vi "Run_VI_Named_specific.vi"(8 "Run VI Named String":string, 10 "Earlier Filenames":path[](array[path]), 11 "Multi Run Row":T1 {"Carrier_2 Q (l/min)" format="%#.2f"; "Row Duration (mins)" format="%#.1f"; "Row No" min=0; "Trace Gas Concentration (%)" min=0.0 format="%#_4f"; "Carrier_1 Q (l/min)" format="%#.2f"; "Tunnel Speed" format="%#.2f"; "Start X" format="%#.2f"; "Start Y" format="%#.2f"; "Start Z" format="%#.2f"; "End X" format="%#.2f"; "End Y" format="%#.2f"; "End Z" format="%#.2f"; "Averaging time (min)" min=0.0 format="%#.2f"}) -> (0 "Scalable Time (Sec)":dbl format="%.2f", 1 "Fixed Time (Sec)":dbl format="%.2f", 2 "Channel Names":string[](array[string]), 3 "Checks":string[](array[string]), 4 "Error String":string, 5 "Check Meas Setup?":bool, 6 "Check for start NaNs?":bool)   [LabVIEW 2015]
uses:
  Gen Trav/Traverse_cluster.ctl
  Gen Trav/Spacing.ctl
  Controls/Multi_run_mode.ctl
  Globals/Preference_global.vi
panel:
  # "X           Y            Z"
  # "Start"
  # "End"
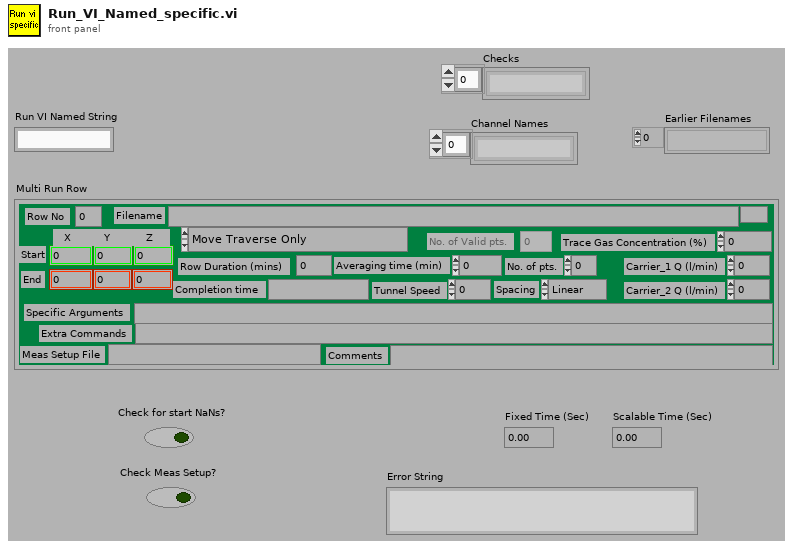
[diagram p1: front panel]
types:
  T1 = typedef "Traverse_cluster.ctl" = cluster{"Start X":sgl, "Start Y":sgl, "Start Z":sgl, "End X":sgl, "End Y":sgl, "End Z":sgl, "No. of pts.":i32, "Spacing":T2, "Filename":path, "Tunnel Speed":dbl, "Averaging time (min)":dbl, "Extra Commands":string, "Carrier_1 Q (l/min)":dbl, "Carrier_2 Q (l/min)":dbl, "Trace Gas Concentration (%)":dbl, "Specific Arguments":string, "Comments":string, "Row No":i32, "Row Type Selector":T3, "Completion time":string, "Row Duration (mins)":dbl, "No. of Valid pts.":i32, "Meas Setup File":string}
  T2 = typedef "Spacing.ctl" = enum16{"Linear", "Log", "Gauss", "Specified", "N/A"}
  T3 = typedef "Multi_run_mode.ctl" = enum16{"Move Traverse Only", "Set Tunnel Speed Only", "Set Source Only", "Set Measurement Conditions", "Single Measurement", "Vertical Profile", "Lateral Profile", "Longitudinal Profile", "Explore Volume", "Multi-Axis Profile", "Auto Calibrate", "Meas Fast FID Bkgnd", "Check Beam Power", "Scanning Valve Measurement", "Run VI Named:", "Set ADAM Ch", "Wait (minutes)", "Send Message", "Synchronize With:", "Fall Back to this Row", "Turn Off Row Repeating", "Blank Row", "Traverse 3D Volume"}
  T4 = typedef "Beam_Type.ctl" = u16
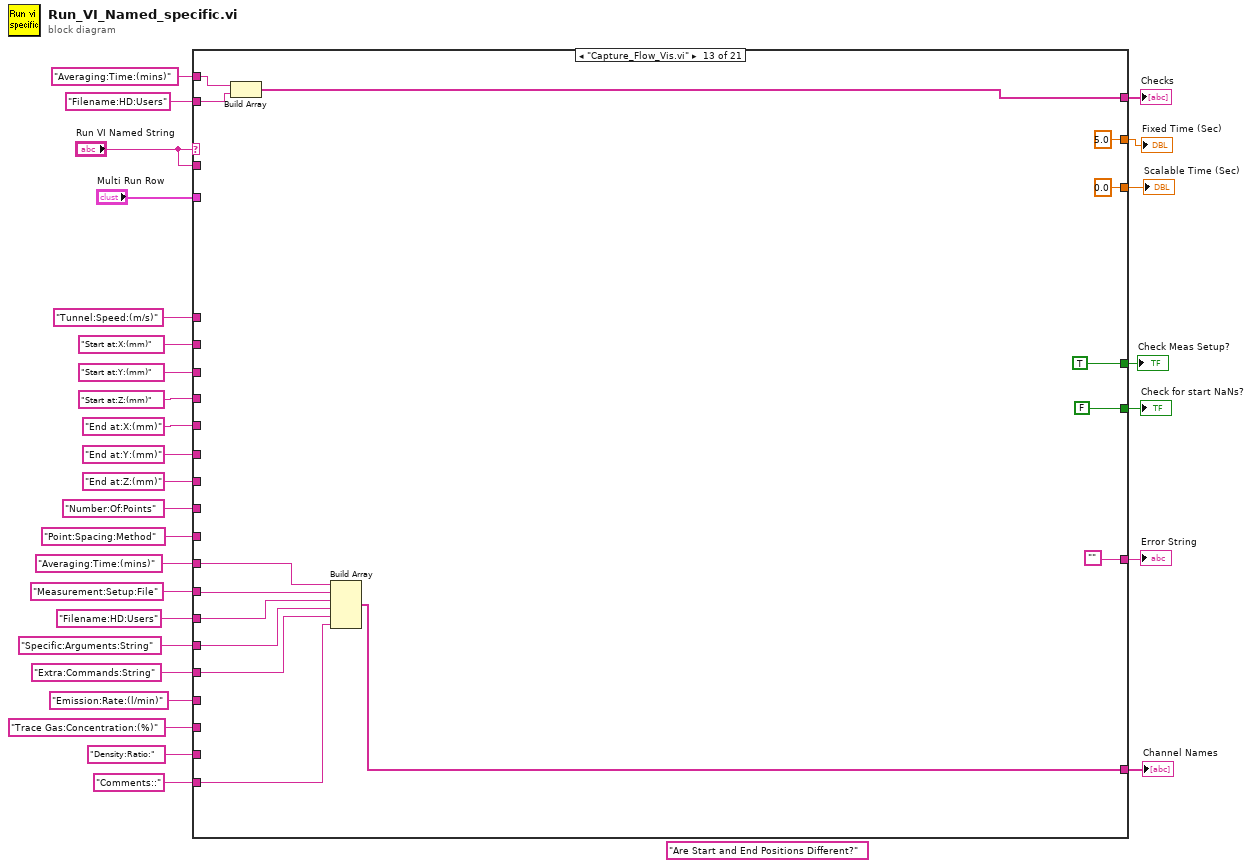
[diagram p0: block diagram]
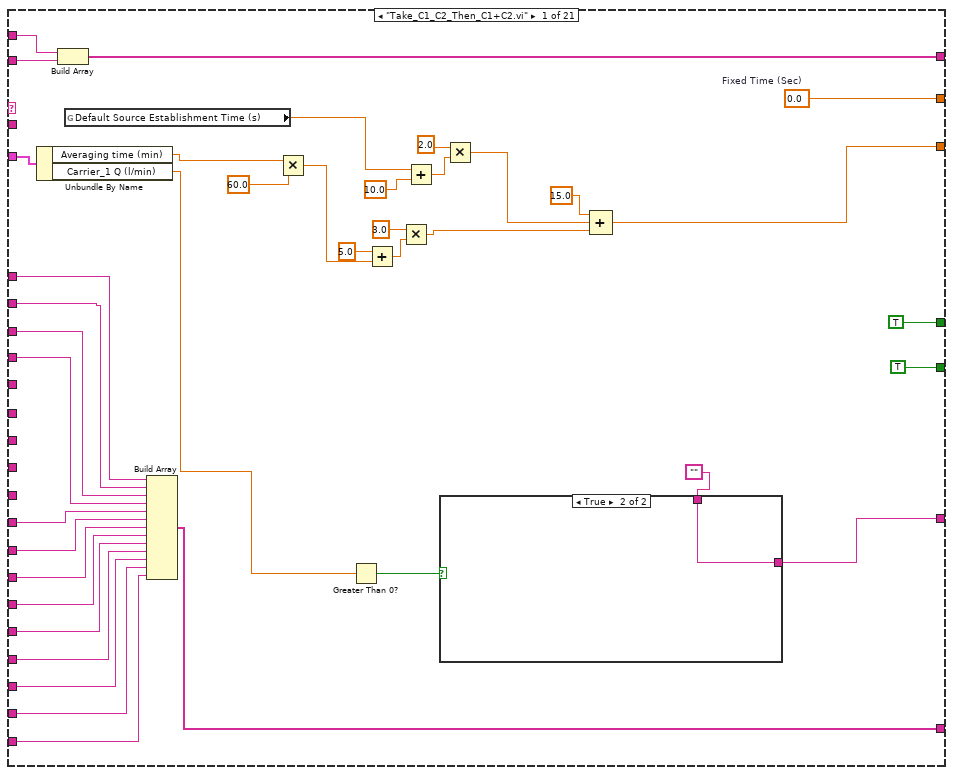
[diagram p2: hidden frame]
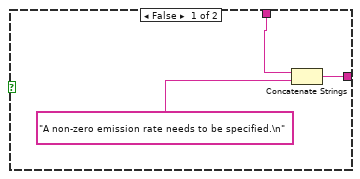
[diagram p3: hidden frame]
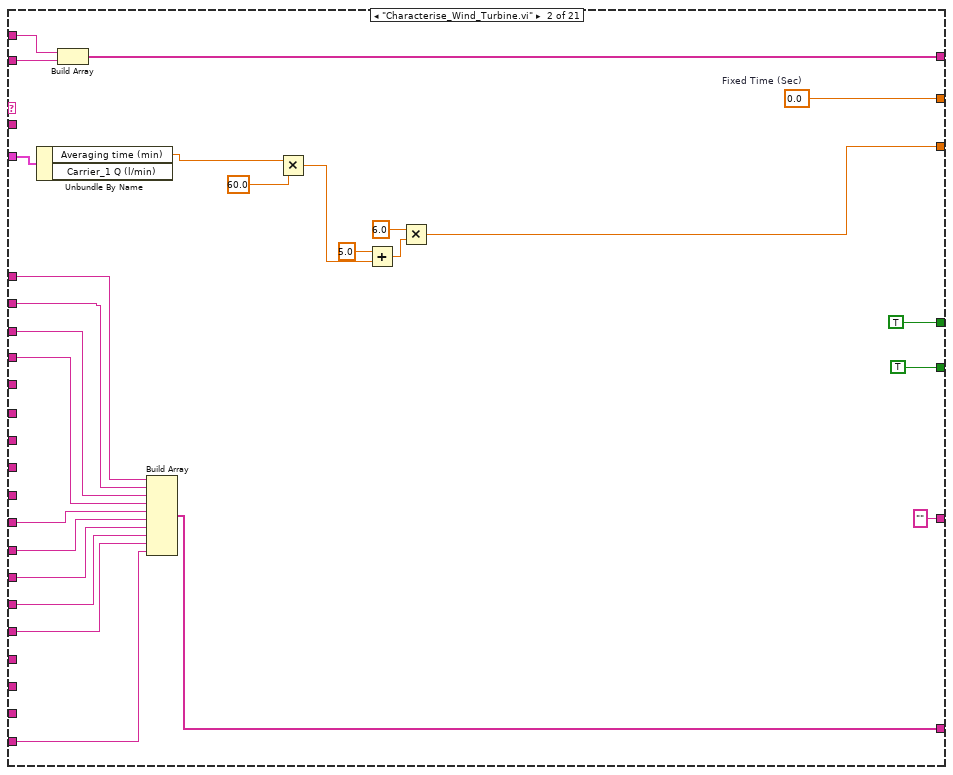
[diagram p4: hidden frame]
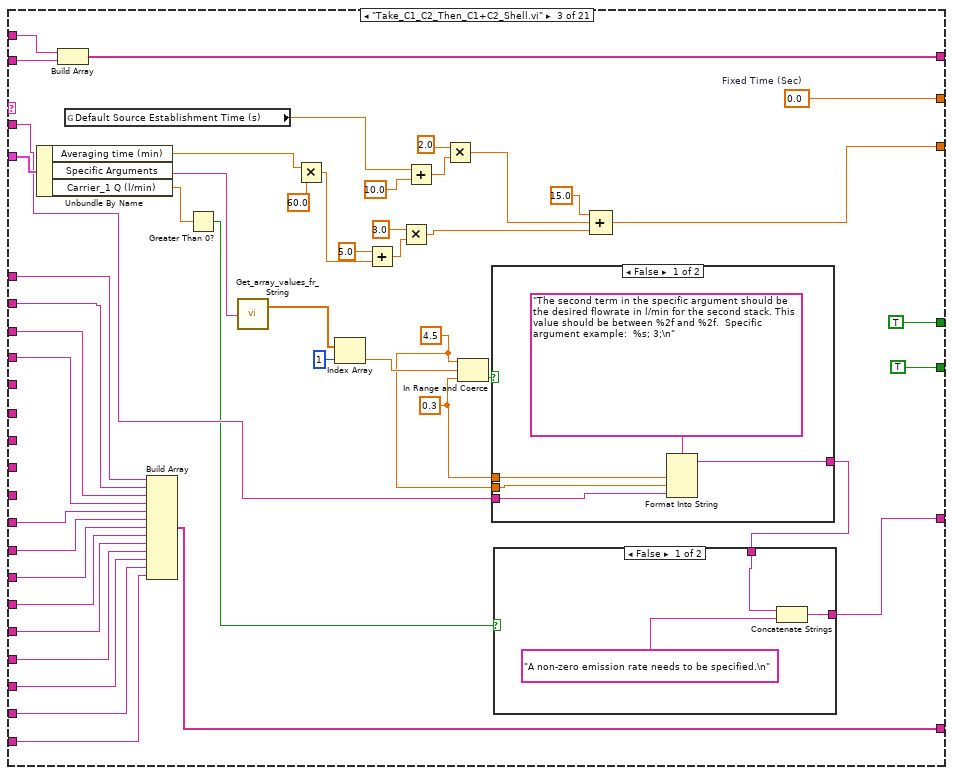
[diagram p5: hidden frame]
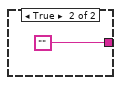
[diagram p7: hidden frame]
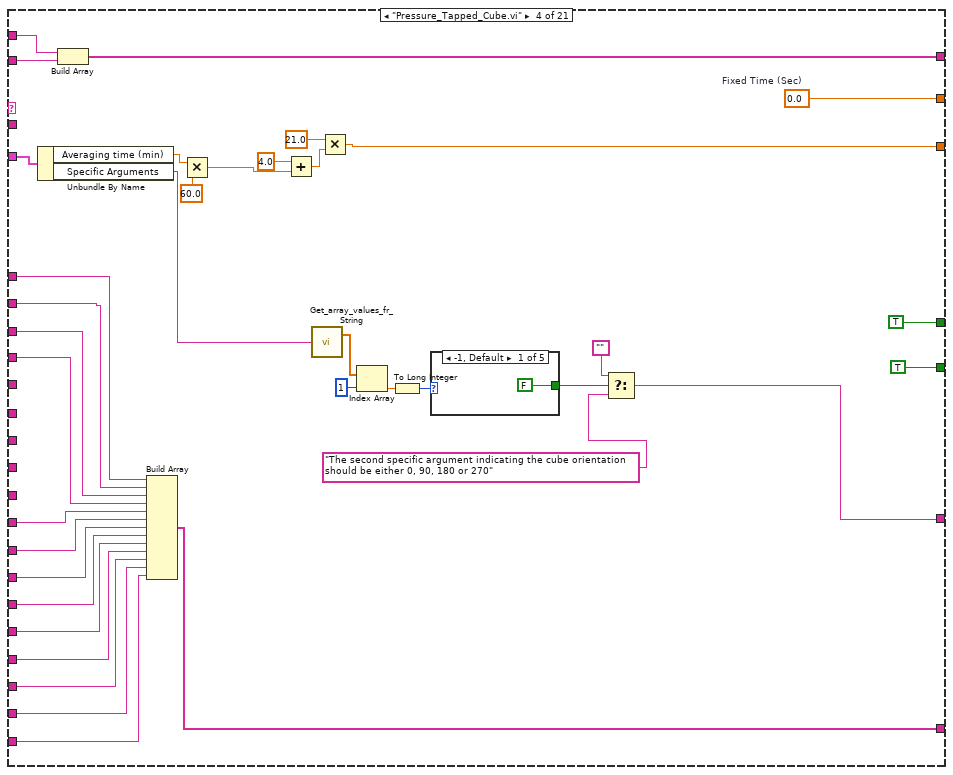
[diagram p8: hidden frame]
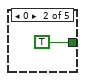
[diagram p9: hidden frame]
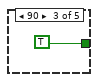
[diagram p10: hidden frame]
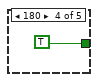
[diagram p11: hidden frame]
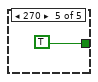
[diagram p12: hidden frame]
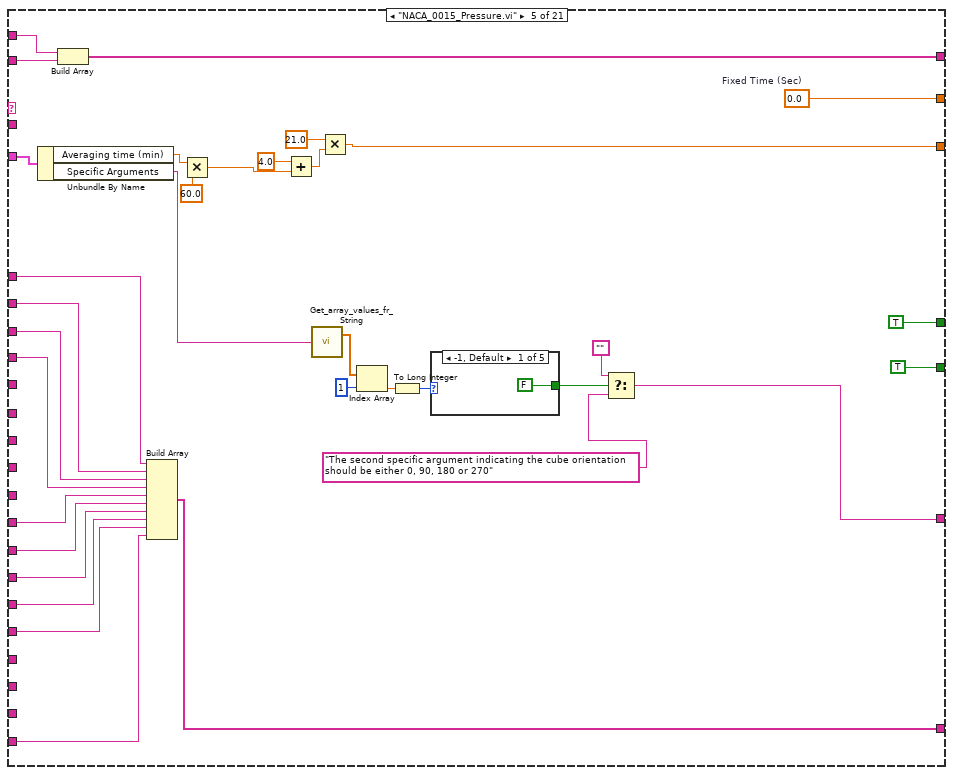
[diagram p13: hidden frame]
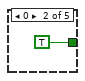
[diagram p14: hidden frame]
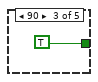
[diagram p15: hidden frame]
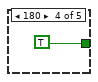
[diagram p16: hidden frame]
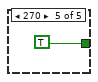
[diagram p17: hidden frame]
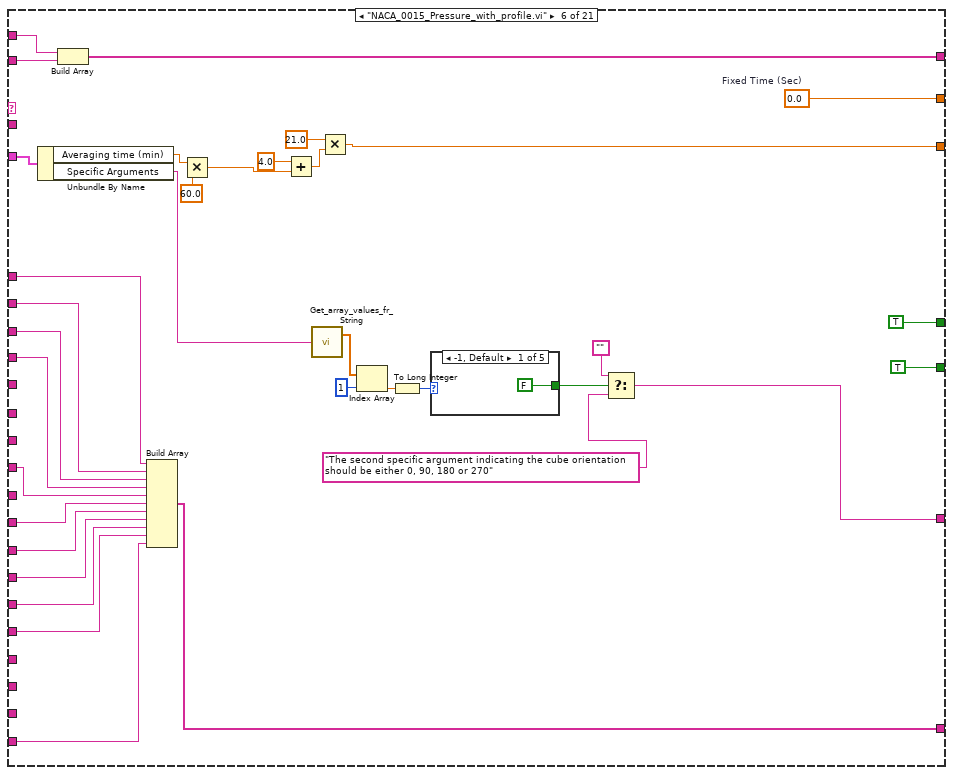
[diagram p18: hidden frame]
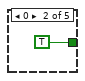
[diagram p19: hidden frame]
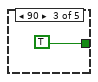
[diagram p20: hidden frame]
diagram:
  (unwired) "Are Start and End Positions Different?" ("Label for value")
  n1 = case shown="\"Capture_Flow_Vis.vi\"" "Run VI Named String" {
    tunnel: "Multi Run Row" -> [w68 w98 w145 w192 w231 w271 w314 w321 _ w376 _ _ _ _ w456 w480 _ _ w527 w556 w582]
    tunnel: [w67 w97 w144 w191 w230 w270 w313 w355 w371 w386 0.0 ("Fixed Time (Sec)") 5.0 ("Fixed Time (Sec)") 5.0 ("Fixed Time (Sec)") 5.0 ("Fixed Time (Sec)") 5.0 ("Fixed Time (Sec)") 5.0 ("Fixed Time (Sec)") 40.0 ("Fixed Time (Sec)") 40.0 ("Fixed Time (Sec)") w521 w548 w581] -> w28
    tunnel: [w53 w74 w130 w165 w210 w250 w295 w319 60.0 ("value") 0.0 ("value") 6.0 ("value") 0.0 ("value") 0.0 ("value") 0.0 ("value") 0.0 ("value") 0.0 ("value") 0.0 ("value") 0.0 ("value") w522 w555 40.0 ("value")] -> w27
    tunnel: "Averaging:Time:(mins)" ("Label for value") -> [w52 w90 w129 w188 w227 w267 w310 w353 w370 _ _ _ w428 _ _ _ _ _ _ _ _]
    tunnel: "Filename:HD:Users" ("Label for value") -> [w51 w89 w128 w187 w226 w266 w309 w352 w369 _ _ _ w426 _ _ _ _ _ _ _ _]
    tunnel: [TRUE TRUE TRUE TRUE TRUE TRUE FALSE TRUE TRUE FALSE FALSE FALSE FALSE FALSE FALSE FALSE FALSE FALSE FALSE FALSE TRUE] -> w24
    tunnel: [TRUE TRUE TRUE TRUE TRUE TRUE TRUE TRUE TRUE FALSE FALSE FALSE TRUE FALSE FALSE FALSE FALSE FALSE FALSE TRUE FALSE] -> w23
    tunnel: [w48 w86 w125 w184 w223 w263 w306 w349 w366 string[] [] string[] [] string[] [] w427 string[] [] string[] [] string[] [] string[] [] string[] [] string[] [] string[] [] string[] []] -> w22
    tunnel: "Tunnel:Speed:(m/s)" ("Label for value") -> [w47 w85 w124 w183 w200 w240 _ w348 _ w377 w400 _ _ _ _ _ _ _ _ w535 _]
    tunnel: "Start at:X:(mm)" ("Label for value") -> [w46 w84 w123 w182 w199 w239 _ w347 w365 _ w409 _ _ _ _ w478 w497 w505 _ _ w578]
    tunnel: "Start at:Y:(mm)" ("Label for value") -> [w45 w83 w122 w181 w198 w238 _ w346 w364 _ w408 _ _ _ _ w477 _ w508 _ _ w577]
    tunnel: "Start at:Z:(mm)" ("Label for value") -> [w44 w82 w121 w180 w222 w262 _ w345 w363 _ w407 _ _ _ _ w476 _ _ _ _ w576]
    tunnel: "Averaging:Time:(mins)" ("Label for value") -> [w43 w81 w120 w179 w221 w261 w291 w344 _ _ w399 _ w430 _ _ _ _ _ _ w544 _]
    tunnel: "Measurement:Setup:File" ("Label for value") -> [w42 w80 w119 w178 w220 w260 w305 w343 w362 _ w395 _ w431 _ _ _ w493 w509 _ w545 _]
    tunnel: "Filename:HD:Users" ("Label for value") -> [w41 w79 w118 w177 w219 w259 w304 w342 _ _ w401 _ w429 _ w457 w474 _ _ _ w546 _]
    tunnel: "Specific:Arguments:String" ("Label for value") -> [w40 w78 w117 w176 w218 w258 w303 w341 w361 w383 w394 w423 w438 w448 w464 w475 w494 w510 w532 w547 w564]
    tunnel: "Extra:Commands:String" ("Label for value") -> [w39 w77 w116 w175 w217 w257 w302 w340 w360 w382 w393 w422 w437 w447 w463 w488 w495 w511 w531 w560 w563]
    tunnel: "Emission:Rate:(l/min)" ("Label for value") -> [w38 _ w115 w174 _ _ _ w339 _ _ w398 _ _ _ _ _ _ _ _ _ _]
    tunnel: "Trace Gas:Concentration:(%)" ("Label for value") -> [w37 _ w114 w173 _ _ _ w338 _ _ w397 _ _ _ _ _ _ _ _ _ _]
    tunnel: "Density:Ratio:" ("Label for value") -> [w36 _ w113 w172 _ _ _ w337 _ _ w396 _ _ _ _ _ _ _ _ _ _]
    tunnel: "Comments::" ("Label for value") -> [w35 w76 w112 w171 w216 w256 w301 w336 w359 w381 w392 w421 w436 w446 w462 w487 w496 w512 w530 w559 w572]
    tunnel: [w34 w75 w111 w170 w215 w255 w300 w335 w358 w380 w391 w420 w435 w445 w461 w486 w502 w517 w529 w558 w575] -> w8
    tunnel: [w32 "" ("Error Comments") w99 w156 w201 w241 w293 w318 "" w372 "" "" "" "" w452 "" "" "" w520 w550 w566] -> w7
    tunnel: "End at:X:(mm)" ("Label for value") -> [_ _ _ _ _ _ _ w317 _ _ w406 _ _ _ _ _ _ w507 _ _ w573]
    tunnel: "End at:Y:(mm)" ("Label for value") -> [_ _ _ _ _ _ _ w316 _ _ w405 _ _ _ _ _ _ w506 _ _ _]
    tunnel: "End at:Z:(mm)" ("Label for value") -> [_ _ _ _ _ _ _ w315 _ _ w404 _ _ _ _ _ _ _ _ _ _]
    tunnel: "Run VI Named String" -> [_ _ w105 _ _ _ _ _ _ _ _ _ _ _ _ _ _ _ _ _ _]
    tunnel: "Number:Of:Points" ("Label for value") -> [_ _ _ _ _ w237 w292 _ _ _ w403 _ _ _ _ _ _ _ _ _ _]
    tunnel: "Point:Spacing:Method" ("Label for value") -> [_ _ _ _ _ _ w290 _ _ _ w402 _ _ _ _ _ _ _ _ _ _]
    frame "Take_C1_C2_Then_C1+C2.vi" {
      w67 = 0.0  # Fixed Time (Sec)
      n2 = Unbundle By Name(w68) -> ("Averaging time (min)"=w56:dbl, "Carrier_1 Q (l/min)"=w31:dbl)
      n3 = Build Array(w52, w51) -> (w48:string[])
      n4 = global read "Preference_global.vi" "Default Source Establishment Time (s)"() -> (w57:dbl)
      n5 = Build Array(w47, w46, w45, w44, w43, w42, w41, w40, w39, w38, w37, w36, w35) -> (w34:string[])
      n6 = Multiply(x=w56, y=60.0) -> (x*y=w54:dbl)
      n7 = Greater Than 0?(x=w31) -> (x > 0?=w30:bool)
      n8 = Add(x=5.0, y=w54) -> (x+y=w60:dbl)
      n9 = Multiply(x=3.0, y=w60) -> (x*y=w64:dbl)
      n10 = Add(x=w57, y=10.0) -> (x+y=w62:dbl)
      n11 = case shown="True" w30 {
        tunnel: "" -> [w70 w72]
        tunnel: [w69 w72] -> w32
        frame False {
          n12 = Concatenate Strings(w70, "A non-zero emission rate needs to be specified.\n") -> (w69:string)
        }
        frame True {
        }
      }
      n13 = Multiply(x=2.0, y=w62) -> (x*y=w65:dbl)
      n14 = Compound Arithmetic op=ADD(15.0 ("value"), w65, w64) -> (w53:dbl)
    }
    frame "Characterise_Wind_Turbine.vi" {
      w97 = 0.0  # Fixed Time (Sec)
      n15 = Unbundle By Name(w98) -> ("Averaging time (min)"=w93:dbl)  [unwired: 1 out]
      n16 = Build Array(w90, w89) -> (w86:string[])
      n17 = Build Array(w85, w84, w83, w82, w81, w80, w79, w78, w77, w76) -> (w75:string[])
      n18 = Multiply(x=w93, y=60.0) -> (x*y=w91:dbl)
      n19 = Add(x=5.0, y=w91) -> (x+y=w96:dbl)
      n20 = Multiply(x=6.0, y=w96) -> (x*y=w74:dbl)
    }
    frame "Take_C1_C2_Then_C1+C2_Shell.vi" {
      w103 = 4.5 ("upper limit")
      w104 = 0.3 ("lower limit")
      w144 = 0.0  # Fixed Time (Sec)
      n21 = Unbundle By Name(w145) -> ("Averaging time (min)"=w133:dbl, "Specific Arguments"=w108:string, "Carrier_1 Q (l/min)"=w102:dbl)
      n22 = Build Array(w129, w128) -> (w125:string[])
      n23 = global read "Preference_global.vi" "Default Source Establishment Time (s)"() -> (w134:dbl)
      n24 = Build Array(w124, w123, w122, w121, w120, w119, w118, w117, w116, w115, w114, w113, w112) -> (w111:string[])
      n25 = Greater Than 0?(x=w102) -> (x > 0?=w101:bool)
      n26 = call "Get_array_values_fr_String.vi"("String Value"=w108) -> ("Numeric Array"=w110:dbl[])  [unwired: 1 out]
      n27 = Multiply(x=w133, y=60.0) -> (x*y=w131:dbl)
      n28 = Index Array(array=w110, index=1) -> (element=w107:dbl)
      n29 = Add(x=5.0, y=w131) -> (x+y=w137:dbl)
      n30 = Multiply(x=3.0, y=w137) -> (x*y=w141:dbl)
      n31 = Add(x=w134, y=10.0) -> (x+y=w139:dbl)
      n32 = Multiply(x=2.0, y=w139) -> (x*y=w142:dbl)
      n33 = In Range and Coerce(upper limit=w103, x=w107, lower limit=w104) -> (In Range?=w106:bool)  [unwired: 1 out]
      n34 = case shown="False" w106 {
        tunnel: [w150 ""] -> w100
        tunnel: w105 -> [w154 _]
        tunnel: w104 -> [w153 _]
        tunnel: w103 -> [w152 _]
        frame False {
          n35 = Format Into String(format string="The second term in the specific argument should be the desired flowrate in l/min for the second stack. This value should be between %2f and %2f.  Specific argument example:  %s; 3;\n", w153, w152, w154) -> (resulting string=w150:string)  [unwired: 2 in, 1 out]
        }
        frame True {
        }
      }
      n36 = case shown="False" w101 {
        tunnel: w100 -> [w147 w149]
        tunnel: [w146 w149] -> w99
        frame False {
          n37 = Concatenate Strings(w147, "A non-zero emission rate needs to be specified.\n") -> (w146:string)
        }
        frame True {
        }
      }
      n38 = Compound Arithmetic op=ADD(15.0 ("value"), w142, w141) -> (w130:dbl)
    }
    frame "Pressure_Tapped_Cube.vi" {
      w191 = 0.0  # Fixed Time (Sec)
      n39 = Unbundle By Name(w192) -> ("Averaging time (min)"=w190:dbl, "Specific Arguments"=w157:string)
      n40 = Build Array(w188, w187) -> (w184:string[])
      n41 = Build Array(w183, w182, w181, w180, w179, w178, w177, w176, w175, w174, w173, w172, w171) -> (w170:string[])
      n42 = Multiply(x=w190, y=60.0) -> (x*y=w166:dbl)
      n43 = Add(x=4.0, y=w166) -> (x+y=w169:dbl)
      n44 = call "Get_array_values_fr_String.vi"("String Value"=w157) -> ("Numeric Array"=w159:dbl[])  [unwired: 1 out]
      n45 = Multiply(x=21.0, y=w169) -> (x*y=w165:dbl)
      n46 = Index Array(array=w159, index=1) -> (element=w160:dbl)
      n47 = To Long Integer(number=w160) -> (32bit integer=w161:i32)
      n48 = case shown="-1, Default" w161 {
        tunnel: [FALSE TRUE TRUE TRUE TRUE] -> w164
        frame -1, Default {
        }
        frame 0 {
        }
        frame 90 {
        }
        frame 180 {
        }
        frame 270 {
        }
      }
      n49 = Select(t="", s=w164, f="The second specific argument indicating the cube orientation should be either 0, 90, 180 or 270") -> (s? t:f=w156:string)
    }
    frame "NACA_0015_Pressure.vi" {
      w230 = 0.0  # Fixed Time (Sec)
      n50 = Unbundle By Name(w231) -> ("Averaging time (min)"=w229:dbl, "Specific Arguments"=w202:string)
      n51 = Build Array(w227, w226) -> (w223:string[])
      n52 = Build Array(w200, w199, w198, w222, w221, w220, w219, w218, w217, w216) -> (w215:string[])
      n53 = Multiply(x=w229, y=60.0) -> (x*y=w211:dbl)
      n54 = Add(x=4.0, y=w211) -> (x+y=w214:dbl)
      n55 = call "Get_array_values_fr_String.vi"("String Value"=w202) -> ("Numeric Array"=w204:dbl[])  [unwired: 1 out]
      n56 = Multiply(x=21.0, y=w214) -> (x*y=w210:dbl)
      n57 = Index Array(array=w204, index=1) -> (element=w205:dbl)
      n58 = To Long Integer(number=w205) -> (32bit integer=w206:i32)
      n59 = case shown="-1, Default" w206 {
        tunnel: [FALSE TRUE TRUE TRUE TRUE] -> w209
        frame -1, Default {
        }
        frame 0 {
        }
        frame 90 {
        }
        frame 180 {
        }
        frame 270 {
        }
      }
      n60 = Select(t="", s=w209, f="The second specific argument indicating the cube orientation should be either 0, 90, 180 or 270") -> (s? t:f=w201:string)
    }
    frame "NACA_0015_Pressure_with_profile.vi" {
      w270 = 0.0  # Fixed Time (Sec)
      n61 = Unbundle By Name(w271) -> ("Averaging time (min)"=w269:dbl, "Specific Arguments"=w242:string)
      n62 = Build Array(w267, w266) -> (w263:string[])
      n63 = Build Array(w240, w239, w238, w262, w237, w261, w260, w259, w258, w257, w256) -> (w255:string[])
      n64 = Multiply(x=w269, y=60.0) -> (x*y=w251:dbl)
      n65 = Add(x=4.0, y=w251) -> (x+y=w254:dbl)
      n66 = call "Get_array_values_fr_String.vi"("String Value"=w242) -> ("Numeric Array"=w244:dbl[])  [unwired: 1 out]
      n67 = Multiply(x=21.0, y=w254) -> (x*y=w250:dbl)
      n68 = Index Array(array=w244, index=1) -> (element=w245:dbl)
      n69 = To Long Integer(number=w245) -> (32bit integer=w246:i32)
      n70 = case shown="-1, Default" w246 {
        tunnel: [FALSE TRUE TRUE TRUE TRUE] -> w249
        frame -1, Default {
        }
        frame 0 {
        }
        frame 90 {
        }
        frame 180 {
        }
        frame 270 {
        }
      }
      n71 = Select(t="", s=w249, f="The second specific argument indicating the cube orientation should be either 0, 90, 180 or 270") -> (s? t:f=w241:string)
    }
    frame "Measure_Synthetic_Jet.vi" {
      w313 = 0.0  # Fixed Time (Sec)
      n72 = Unbundle By Name(w314) -> ("Averaging time (min)"=w312:dbl, "Specific Arguments"=w294:string)
      n73 = Build Array(w310, w309) -> (w306:string[])
      n74 = Build Array(w292, w290, w291, w305, w304, w303, w302, w301) -> (w300:string[])
      n75 = Multiply(x=w312, y=60.0) -> (x*y=w296:dbl)
      n76 = Add(x=4.0, y=w296) -> (x+y=w299:dbl)
      n77 = call "Get_array_values_fr_String.vi"("String Value"=w294) -> ("String array"=w289:string[])  [unwired: 1 out]
      n78 = Multiply(x=21.0, y=w299) -> (x*y=w295:dbl)
      n79 = Index Array(array=w289, index #1=1 ("index")) -> (element #1=w284:string, element #2=w282:string, element #3=w281:string, element #4=w278:string)  [unwired: 3 in]
      n80 = Empty String/Path?(string/path=w278) -> (empty?=w277:bool)
      n81 = Empty String/Path?(string/path=w282) -> (empty?=w279:bool)
      n82 = Empty String/Path?(string/path=w284) -> (empty?=w283:bool)
      n83 = Empty String/Path?(string/path=w281) -> (empty?=w280:bool)
      n84 = Compound Arithmetic op=OR(w283, w279, w280, w277) -> (w287:bool)
      n85 = Select(t="The second, third and fourth specific argument indicate the min frequency, max frequency, the number of bins to use in the phase average and the target amplitude.  Set the target optimisation target value to -1 if you do not want any optimisation. Example: Measure_Synthetic_Jet.vi; 100; 1000; 50; 0.02", s=w287, f="") -> (s? t:f=w293:string)
    }
    frame "Take_Data_on_the_Move.vi" {
      w355 = 0.0  # Fixed Time (Sec)
      n86 = Build Array(w353, w352) -> (w349:string[])
      n87 = Build Array(w348, w347, w346, w345, w317, w316, w315, w344, w343, w342, w341, w340, w339, w338, w337, w336) -> (w335:string[])
      n88 = Unbundle By Name(w321) -> ("Averaging time (min)"=w320:dbl, "Start X"=w322:sgl, "Start Y"=w323:sgl, "Start Z"=w324:sgl, "End X"=w325:sgl, "End Y"=w326:sgl, "End Z"=w327:sgl)
      n89 = Build Array(w322, w323, w324) -> (w329:sgl[])
      n90 = Build Array(w325, w326, w327) -> (w328:sgl[])
      n91 = Multiply(x=w320, y=60.0) -> (x*y=w333:dbl)
      n92 = Not Equal?(x=w329, y=w328) -> (x != y?=w332:bool)
      n93 = Select(t="", s=w332, f="The Start and End positions must not be the same.\n" ("Format String")) -> (s? t:f=w318:string)
      n94 = Add(x=10.0, y=w333) -> (x+y=w319:dbl)
    }
    frame "Check_FID_Response.vi" {
      w371 = 0.0  # Fixed Time (Sec)
      n95 = Build Array(w370, w369) -> (w366:string[])
      n96 = Build Array(w365, w364, w363, w362, w361, w360, w359) -> (w358:string[])
    }
    frame "Return_EnFlo_Tunnel_to_Neutral.vi" {
      w373 = 0.4 ("y")
      w386 = 240.0  # Fixed Time (Sec)
      n97 = Unbundle By Name(w376) -> ("Tunnel Speed"=w375:dbl)
      n98 = Build Array(w377, w383, w382, w381) -> (w380:string[])
      n99 = Greater?(x=w375, y=w373) -> (0:w374:bool)
      n100 = case shown="True" w374 {
        tunnel: w373 -> [w389 _]
        tunnel: [w387 ""] -> w372
        frame False {
          n101 = Format Into String(format string="The Tunnel speed must be greater than %.1f", w389) -> (resulting string=w387:string)  [unwired: 2 in, 1 out]
        }
        frame True {
        }
      }
    }
    frame "No Match", Default {
      n102 = Build Array(w409, w408, w407, w406, w405, w404, w403, w402, w401, w400, w399, w393, w394, w398, w397, w396, w392, w395) -> (w391:string[])
    }
    frame "Set_Wind_Turbine_Speed.vi" {
      n103 = Build Array(w423, w422, w421) -> (w420:string[])
    }
    frame "Capture_Flow_Vis.vi" {
      n104 = Build Array(w428, w426) -> (w427:string[])
      n105 = Build Array(w430, w431, w429, w438, w437, w436) -> (w435:string[])
    }
    frame "Shut_down_EnFlo_Tunnel.vi" {
      n106 = Build Array(w448, w447, w446) -> (w445:string[])
    }
    frame "Update_Inlet_Temp_Profile.vi" {
      n107 = Unbundle By Name(w456) -> ("Filename"=w451:path)
      n108 = Build Array(w457, w464, w463, w462) -> (w461:string[])
      n109 = Search 1D Array(1D array="Earlier Filenames", element=w451) -> (index of element=w454:i32)  [unwired: 1 in]
      n110 = case shown="0, Default" w454 {
        tunnel: w451 -> [_ w473]
        tunnel: [TRUE ("exists?") w472] -> w453
        frame 0, Default {
        }
        frame -1 {
          n111 = call "Does_file_exist_(simple).vi"("Pathname"=w473) -> ("exists?"=w472:bool)
        }
      }
      n112 = case shown="False" w453 {
        tunnel: [w467 ""] -> w452
        tunnel: w451 -> [w469 _]
        frame False {
          n113 = Format Into String(format string="Cannot find Filename%s", w469) -> (resulting string=w467:string)  [unwired: 2 in, 1 out]
        }
        frame True {
        }
      }
    }
    frame "Datum_Image_Calibration.vi" {
      n114 = Unbundle By Name(w480) -> ("Filename"=w479:path)
      n115 = Build Array(w478, w477, w476, w474, w475, w488, w487) -> (w486:string[])
      n116 = call "Does_file_exist_(simple).vi"("Pathname"=w479) -> ("exists?"=w481:bool)
      n117 = case shown="False" w481 {
        tunnel: w479 -> [w492 _]
        frame False {
          n118 = Write to Text File(file (use dialog)=w492, text="Created so that multirun checker is happy that the file exists") -> ()  [unwired: 2 in, 3 out]
        }
        frame True {
        }
      }
    }
    frame "EnFlo_Turntable_Control.vi" {
      n119 = Build Array(w497, w493, w494, w495, w496) -> (w502:string[])
    }
    frame "Plot_Rectangle.vi" {
      n120 = Build Array(w505, w508, w507, w506, w509, w510, w511, w512) -> (w517:string[])
    }
    frame "Find_Beam_Max_Pos.vi" {
      w526 = 240.0  # Fixed Time (Sec)
      w522 = 0.0  # Scalable Time (Sec)
      n121 = Unbundle By Name(w527) -> ("Specific Arguments"=w523:string)
      n122 = Build Array(w532, w531, w530) -> (w529:string[])
      n123 = call "Get_Beam_names.vi"("String Value"=w523) -> ("Beam Array"=w524:T4[], "Error Comments"=w520:string)  [unwired: 1 out]
      n124 = Array Size(array=w524) -> (size(s)=w525:i32)
      n125 = Multiply(x=w526, y=w525) -> (x*y=w521:dbl)
    }
    frame "Find_Max_Value.vi" {
      w548 = 240.0  # Fixed Time (Sec)
      w555 = 0.0  # Scalable Time (Sec)
      n126 = Unbundle By Name(w556) -> ("Specific Arguments"=w553:string)
      n127 = Build Array(w535, w544, w545, w546, w547, w560, w559) -> (w558:string[])
      n128 = call "Get_array_values_fr_String.vi"("String Value"=w553) -> ("String array"=w554:string[])  [unwired: 1 out]
      n129 = Index Array(array=w554) -> (element #2=w552:string, element #3=w543:string, element #4=w537:string, element #5=w536:string)  [unwired: 5 in, 1 out]
      n130 = Empty String/Path?(string/path=w536) -> (empty?=w539:bool)
      n131 = Empty String/Path?(string/path=w552) -> (empty?=w542:bool)
      n132 = Empty String/Path?(string/path=w543) -> (empty?=w541:bool)
      n133 = Empty String/Path?(string/path=w537) -> (empty?=w538:bool)
      n134 = Compound Arithmetic op=OR(w542, w541, w538, w539) -> (w540:bool)
      n135 = Select(t="The second argument should be contain the fixed axis, followed by the search step in mm, the measurement channel to use for the survey and finally the data type you would like to measure, for example: Z Axis; 0.75; 2; uw/u'w'", s=w540, f="" ("Error Comments")) -> (s? t:f=w550:string)
    }
    frame "Move_Twin_Stacks.vi" {
      w581 = 0.0  # Fixed Time (Sec)
      n136 = Unbundle By Name(w582) -> ("End X"=w569:sgl)
      n137 = Build Array(w578, w577, w576, w573, w564, w563, w572) -> (w575:string[])
      n138 = Absolute Value(x=w569) -> (abs(x)=w568:sgl)
      n139 = Greater Than 0?(x=w568) -> (x > 0?=w571:bool)
      n140 = Select(t="", s=w571, f="The \"End X\" is the x seperation distance of the moving source from the reference.") -> (s? t:f=w566:string)
    }
  }
  "Fixed Time (Sec)" <- w28
  "Scalable Time (Sec)" <- w27
  "Check Meas Setup?" <- w23
  "Error String" <- w7
  "Check for start NaNs?" <- w24
  "Checks" <- w22
  "Channel Names" <- w8
